vi "Edit calibration.vi"(2 "Ports":T1, 3 "Data Display":T3 {"average data rate (Hz)" format="%.2f"; "Min Voltage" format="%.3f"; "Max Voltage" format="%.3f"; "Mean (Volts)" format="%.5f"; "Mean (scaled)" format="%.2f"}, 4 "Index":u32) -> ()   [LabVIEW 2015]
uses:
  conversion.ctl
  DAQ configuration/scale type.ctl
  correspondence table.ctl
  pH/pH scale.ctl
  Dissolved Oxygen/DO scale.ctl
  Spectrophotometer/Photometer calibration data.ctl
  calibrator graph.ctl
  DAQ configuration/Sensor array.ctl
  DAQ configuration/channel identifier.ctl
  DAQ configuration/Sensor buffer command.ctl
  <vilib>/Analysis/1siggen.llb/Ramp Pattern by Samples.vi
  <vilib>/Analysis/NI_AALBase.lvlib
panel:
  out "Calibration Graph":cluster{"Ramp Pattern":dbl[], sgl[]}(graph)
  out "Calibration in":T4 {"D.O."."K" format="%.6f"; "D.O."."Temperature" format="%.2f"; "pH scale"."Buffers"."V/T" format="%.5f"; "pH scale"."Buffers"."Buffer" format="%.2f"; "pH scale"."Temperature" format="%.2f"; "offset (physical units)" format="%.5f"; "correspondence table"."volts" format="%.4f"; "correspondence table"."physical units" format="%.4f"; "second channel" min=-1; "offset (volts)" format="%.5f"; "conversion matrix" format="%.4e"}
  in  "Cancel Button":bool
  in  "OK Button":bool
  in  "Calibration":T4 {"D.O."."K" format="%.6f"; "D.O."."Temperature" format="%.2f"; "pH scale"."Buffers"."V/T" format="%.5f"; "pH scale"."Buffers"."Buffer" format="%.2f"; "pH scale"."Temperature" format="%.2f"; "offset (physical units)" format="%.5f"; "correspondence table"."volts" format="%.4f"; "correspondence table"."physical units" format="%.4f"; "second channel" min=-1; "offset (volts)" format="%.5f"; "conversion matrix" format="%.4e"}
  # "V"
  # "V"
  # "C"
  # "kPa"
  # "C"
  # "C"
  # "kPa"
  # "C"
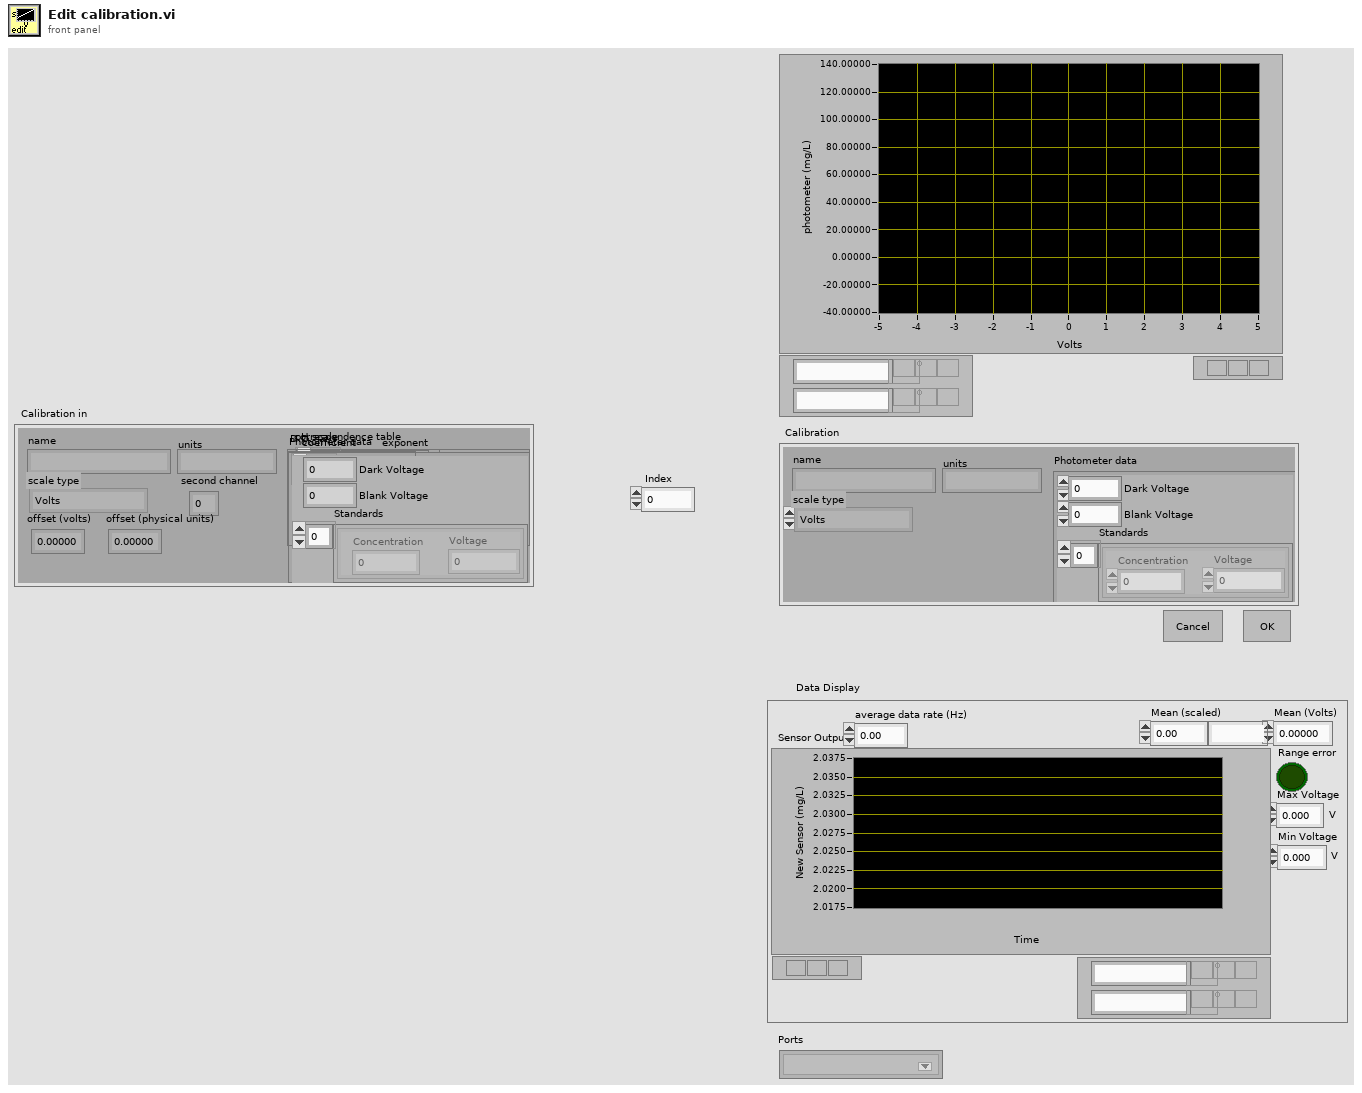
[diagram p1: front panel]
types:
  T1 = typedef "Sensor array.ctl" = T2[]
  T2 = typedef "channel identifier.ctl" = u16
  T3 = typedef "calibrator graph.ctl" = cluster{"Range error":bool, "Mean (scaled)":dbl, "Mean (Volts)":dbl, "Max Voltage":dbl, "Min Voltage":dbl, "units":string, "Sensor Output":cluster{dbl[], dbl[]}[], "average data rate (Hz)":dbl}
  T4 = typedef "conversion.ctl" = cluster{"conversion matrix":sgl[][], "units":string, "name":string, "scale type":T5, "offset (volts)":dbl, "second channel":i8, "correspondence table":T6, "offset (physical units)":dbl, "pH scale":T7, "D.O.":T8, "Photometer data":T9}
  T5 = typedef "scale type.ctl" = enum16{"Volts", "Polynomial", "Correspondence Table", "pH", "Dissolved Oxygen", "Quadratic", "Photometer"}
  T6 = typedef "correspondence table.ctl" = cluster{"physical units":dbl, "volts":dbl}[]
  T7 = typedef "pH scale.ctl" = cluster{"Buffers":cluster{"Buffer":dbl, "Calibrated":bool, "V/T":dbl}[], "Temperature":dbl}
  T8 = typedef "DO scale.ctl" = cluster{"Temperature":dbl, "K":dbl, "barometric pressure":dbl}
  T9 = typedef "Photometer calibration data.ctl" = cluster{"Dark Voltage":dbl, "Blank Voltage":dbl, "Standards":cluster{"Concentration":dbl, "Voltage":dbl}[]}
  T10 = typedef "Sensor buffer command.ctl" = enum16{"read average", "read recent", "read all", "write", "set buffer size", "Read channel config", "Write channel config", "clear"}
  T11 = typedef "Channel config.ctl" = cluster{"Channel Indices":T2[], "AI Max voltage":dbl[], "Calibration matrix":T12}
  T12 = typedef "calib array.ctl" = T4[]
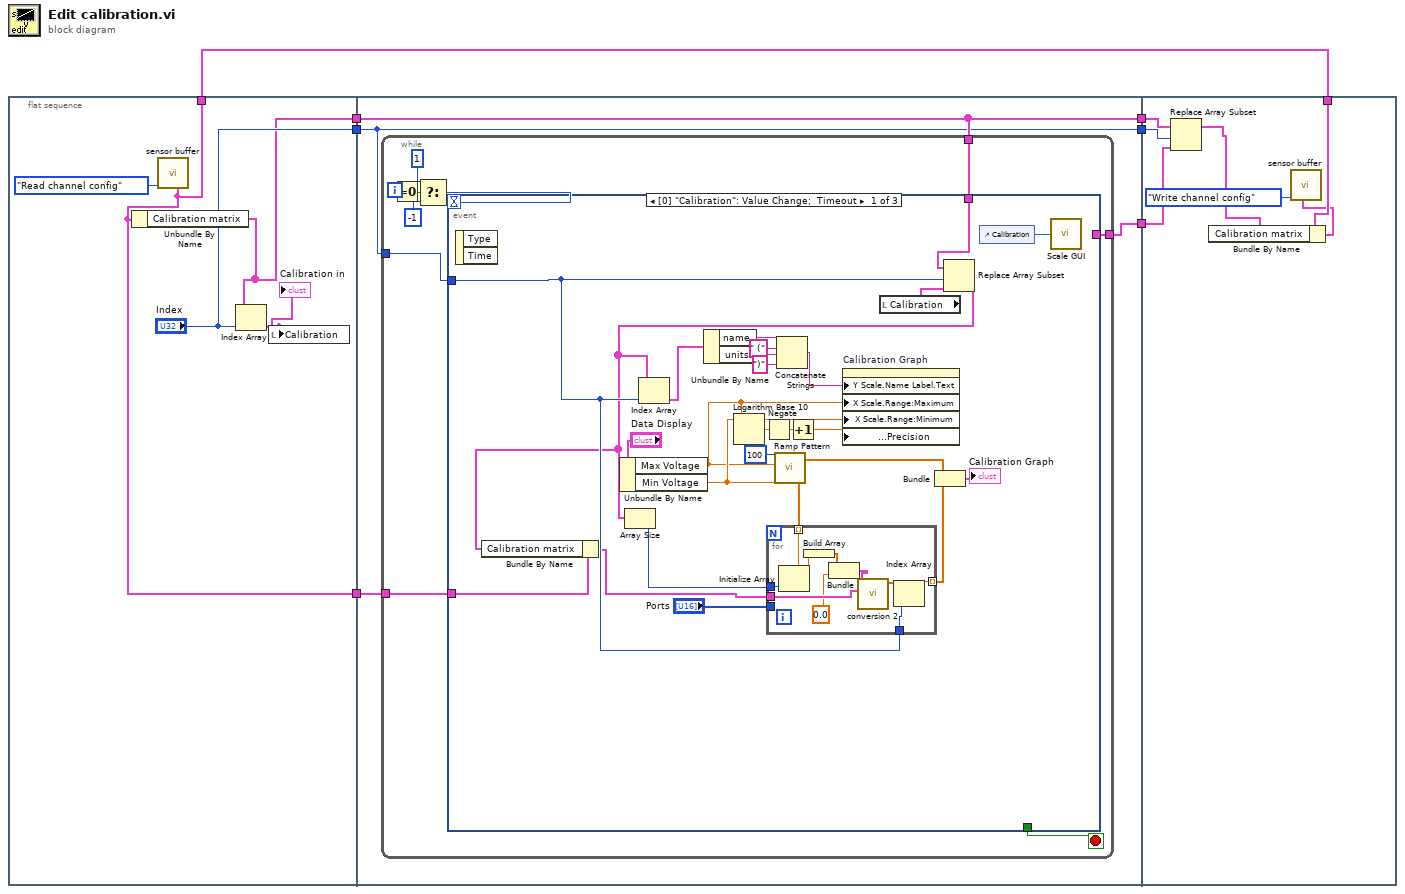
[diagram p0: block diagram]
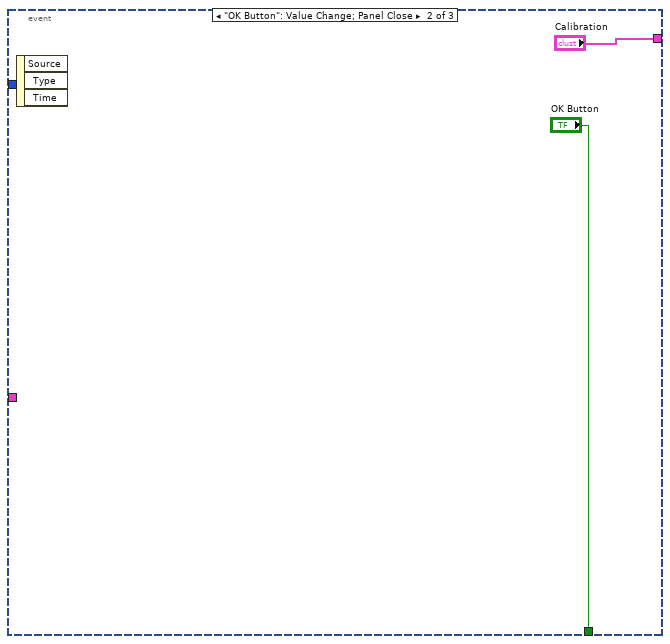
[diagram p2: hidden frame]
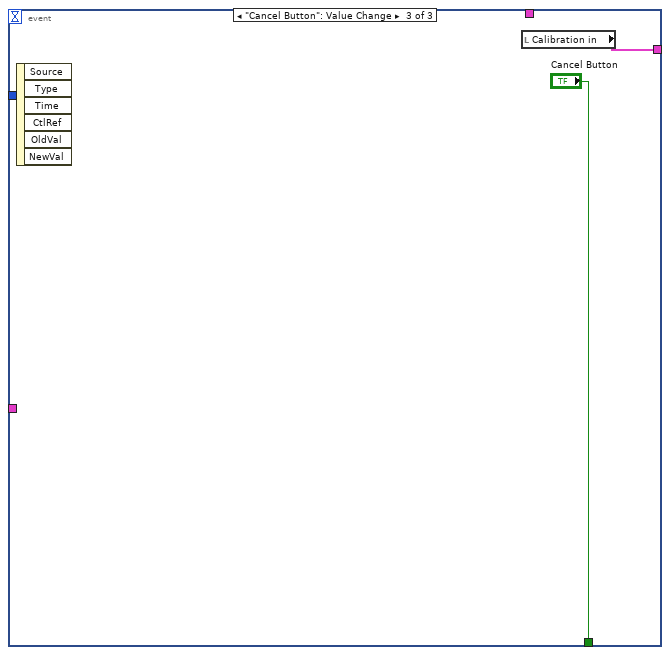
[diagram p3: hidden frame]
diagram:
  n1 = flat-sequence {
    tunnel: [w9] -> w6
    tunnel: ["Index"] -> w4
    tunnel: [w8] -> w2
    tunnel: [w8] -> w1
    tunnel: [w15] -> w7
    tunnel: w6 -> [w15]
    tunnel: [w14] -> w5
    tunnel: w4 -> [w14]
    tunnel: [w16] -> w3
    tunnel: w1 -> [w13]
    tunnel: w7 -> [w71]
    tunnel: w5 -> [w70]
    tunnel: w3 -> [w69]
    tunnel: w2 -> [w66]
    frame #0 {
      n2 = call "sensor buffer.vi"("command"=Sensor_buffer_command."Read channel config") -> ("Channel Config out"=w8:T11)  [unwired: 6 in, 4 out]
      n3 = Unbundle By Name(w8) -> ("Calibration matrix"=w9:T12)
      n4 = Index Array(array=w9, index="Index") -> (element=w12:T4)
      "Calibration in" <- w12
      n5 = local write "Calibration"(w12) -> ()
    }
    frame #1 {
      n6 = while {
        tunnel: [w26] -> w16
        tunnel: w15 -> [w19]
        tunnel: w14 -> [w18]
        tunnel: w13 -> [w17]
        i -> [w21]
        stop <- w25 stop-if-true
        n7 = Equal To 0?(x=w21) -> (x = 0?=w20:bool)
        n8 = Select(t=1, s=w20, f=-1) -> (s? t:f=w22:i32)
        n9 = event shown="[0] \"Calibration\": Value Change;  Timeout" {
          selector: _ -> [_ _ _]
          dyn-events: _ -> [_ _ _]
          timeout: w22 -> [_ _ _]
          tunnel: [_ "Calibration" w63] -> w26
          tunnel: [_ "OK Button" "Cancel Button"] -> w25
          tunnel: w19 -> [w49 _ _]
          tunnel: w18 -> [w31 _ _]
          tunnel: w17 -> [w29 _ _]
          event Value Change; Timeout {
            n10 = event-data() -> ()  [unwired: 1 in, 2 out]
            n11 = Unbundle By Name("Data Display") -> ("Max Voltage"=w36:dbl, "Min Voltage"=w38:dbl)
            n12 = Logarithm Base 10(1:w36) -> (0:w37:dbl)
            n13 = Negate(x=w37) -> (-x=w35:dbl)
            n14 = call-poly <vilib>:"Ramp Pattern.vi"("start"=w38, "end"=w36, "samples"=100) -> ("Ramp Pattern"=w46:dbl[])  [unwired: 7 in, 1 out]
            n15 = Increment(x=w35) -> (x+1=w34:dbl)
            n16 = local read "Calibration"() -> (w50:T4)
            n17 = Replace Array Subset(array=w49, new element=w50, index=w31) -> (w28:T12)
            n18 = Bundle By Name(cluster=w29, "Calibration matrix"=w28) -> (w27:T11)
            n19 = Array Size(array=w28) -> (size(s)=w32:i32)
            n20 = Index Array(array=w28, index=w31) -> (element=w44:T4)
            n21 = Unbundle By Name(w44) -> ("name"=w43:string, "units"=w41:string)
            n22 = for {
              tunnel: w46 -> [w55] mode=indexing
              tunnel: [w59] -> w33 mode=indexing
              tunnel: w32 -> [w58]
              tunnel: w31 -> [w57]
              tunnel: "Ports" -> [_]
              tunnel: w27 -> [w56]
              n23 = Initialize Array(w55, w58) -> ()  [unwired: 1 out]
              n24 = Build Array(w55) -> (w54:dbl[])
              n25 = Bundle(w54, 0.0) -> (w52:cluster{dbl[], dbl})  [unwired: 1 in]
              n26 = call "conversion 2.vi"("Channel Config"=w56, "raw Data"=w52) -> ("calibrated data"=w60:sgl[])  [unwired: 7 in, 2 out]
              n27 = Index Array(array=w60, index=w57) -> (element=w59:sgl)
            }
            n28 = Concatenate Strings(w43, " (" ("Substring"), w41, ")" ("Substring")) -> (w39:string)
            n29 = property on="Calibration Graph" class="XYGraph (strict)"("Y Scale.Name Label.Text"=w39, "X Scale.Range:Maximum"=w36, "X Scale.Range:Minimum"=w38, "X Scale.Format & Precision:Precision"=w34) -> ()  [unwired: 2 in, 2 out]
            n30 = Bundle("Ramp Pattern"=w46, w33) -> (→"Calibration Graph":cluster{"Ramp Pattern":dbl[], sgl[]})  [unwired: 1 in]
            n31 = control-ref of="Calibration"() -> (w51:refnum<vi>)
            n32 = call "Scale GUI.vi"("Clust Refnum"=w51) -> ()
          }
          event "OK Button": Value Change; Panel Close {
            n33 = event-data() -> ()  [unwired: 1 in, 3 out]
          }
          event "Cancel Button": Value Change {
            n34 = event-data() -> ()  [unwired: 1 in, 6 out]
            n35 = local read "Calibration in"() -> (w63:T4)
          }
        }
      }
    }
    frame #2 {
      n36 = Replace Array Subset(array=w71, new element=w69, index=w70) -> (w67:T12)
      n37 = Bundle By Name(cluster=w66, "Calibration matrix"=w67) -> (w65:T11)
      n38 = call "sensor buffer.vi"("Channel Config"=w65, "command"=Sensor_buffer_command."Write channel config") -> ()  [unwired: 5 in, 5 out]
    }
  }
